vi "plunge_mode_scaled.vi"() -> ()   [LabVIEW 2019]
uses:
  <userlib>/Nanonis Prog Interface V5/Nanonis Prog Interface.lvlib
  <userlib>/Haptic Prog Interface/Haptic Prog Interface.lvlib
panel:
  out "Zthresh (m)":dbl
  in  "Fine Adj":dbl=1.0
  in  "Rough Adj.":dbl
  out "force":dbl
  out "Z Write (m) 2":dbl
  in  "Z Write?":bool
  in  "Save":bool
  in  "# Sample Points":i32=16384
  out "Signal value":sgl format="%#_6p"
  out "Z Write (m)":dbl
  in  "Upper Limit (mm)":dbl=50.0
  in  "Lower Limit (mm)":dbl=-40.0
  in  "Upper Limit (nm)":dbl=80.0
  in  "Lower Limit (nm)":dbl=79.0
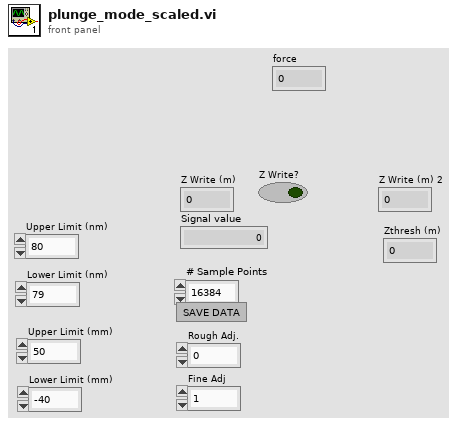
[diagram p1: front panel]
types:
  T1 = cluster{"Fx (N)":dbl, "Fy (N)":dbl, "Fz (N)":dbl}
  T2 = cluster{"x (mm)":dbl, "y (mm)":dbl, "z (mm)":dbl}
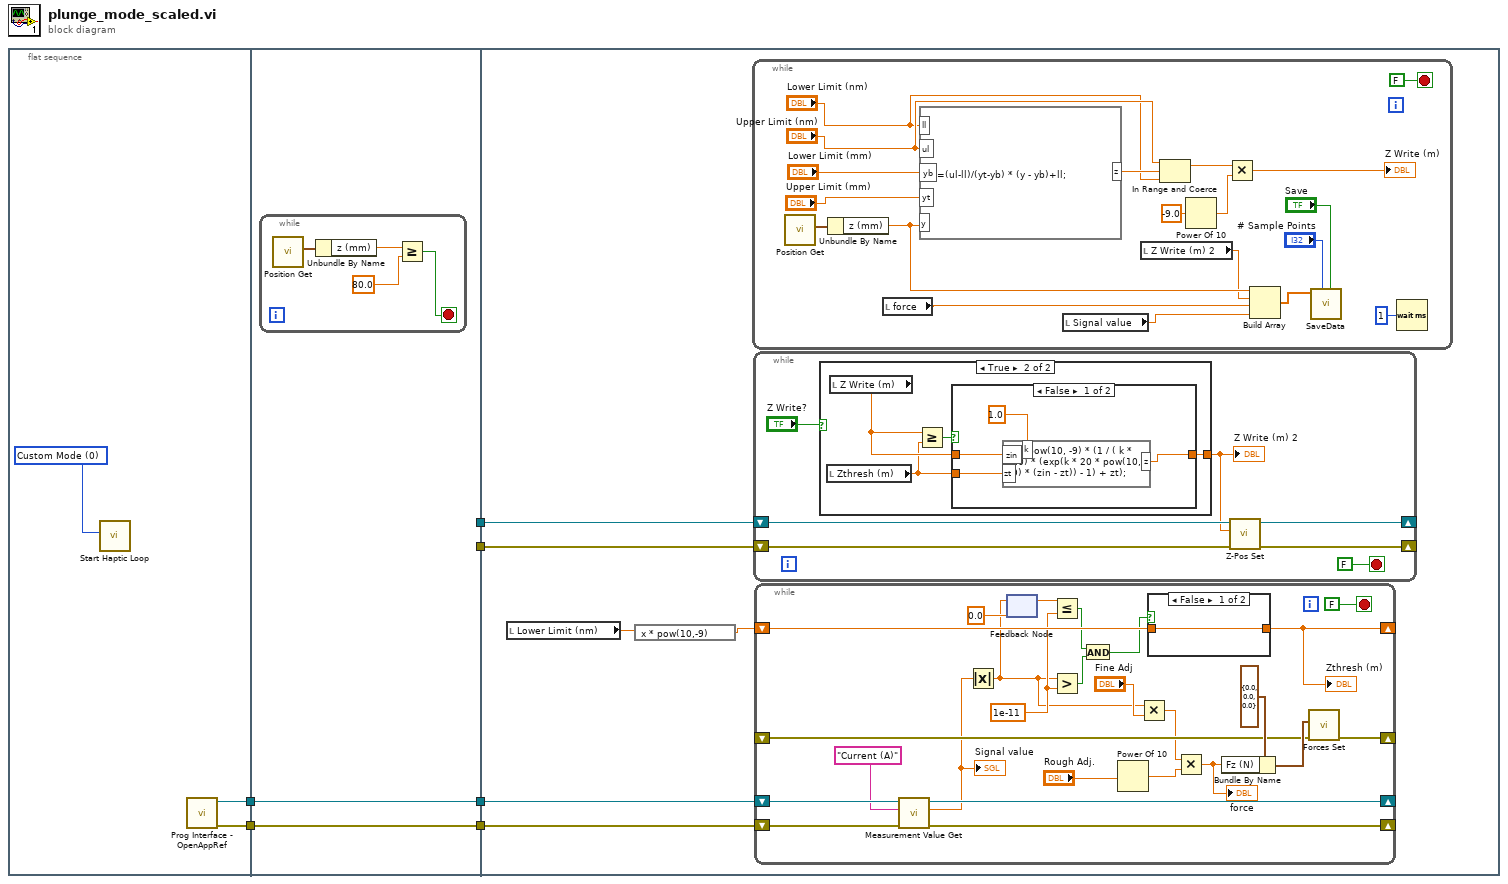
[diagram p0: block diagram]
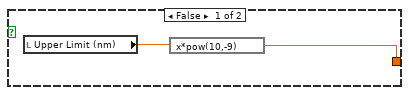
[diagram p2: hidden frame]
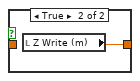
[diagram p4: hidden frame]
diagram:
  n1 = flat-sequence {
    tunnel: [w9] -> w6
    tunnel: [w8] -> w3
    tunnel: [w11] -> w5
    tunnel: [w10] -> w4
    tunnel: [w11] -> w2
    tunnel: [w10] -> w1
    tunnel: w3 -> [w10]
    tunnel: w6 -> [w11]
    tunnel: w5 -> [w21]
    tunnel: w4 -> [w20]
    tunnel: w2 -> [w19]
    tunnel: w1 -> [w18]
    frame #0 {
      w7 = u16 0 items=["Custom Mode", "Read Mode", "Write Mode"] ("Mode Selection")
      n2 = call <userlib>:"Start Haptic Loop.vi"("Mode Selection"=w7) -> ()  [unwired: 10 in, 1 out]
      n3 = call <userlib>:"Prog Interface - OpenAppRef.vi"() -> ("Error out"=w8:errorcluster, "Application reference"=w9:refnum<vi>)  [unwired: 6 in]
    }
    frame #1 {
      n4 = while {
        stop <- w14 stop-if-true
        n5 = call <userlib>:"Position Get.vi"() -> ("Position"=w13:T2)  [unwired: 10 in, 1 out]
        n6 = Unbundle By Name(w13) -> ("z (mm)"=w12:dbl)
        n7 = Greater Or Equal?(x=w12, y=80.0) -> (x >= y?=w14:bool)
      }
    }
    frame #2 {
      n8 = local read "Lower Limit (nm)"() -> (w17:dbl)
      n9 = expression code="x * pow(10,-9)"(w17) -> (w16:dbl)
      n10 = while {
        stop <- FALSE stop-if-true
        n11 = call <userlib>:"Position Get.vi"() -> ("Position"=w71:T2)  [unwired: 10 in, 1 out]
        n12 = Unbundle By Name(w71) -> ("z (mm)"=w70:dbl)
        n13 = local read "force"() -> (w68:dbl)
        n14 = formula code="z =(ul-ll)/(yt-yb) * (y - yb)+ll;"("ll"="Lower Limit (nm)", "ul"="Upper Limit (nm)", "yb"="Lower Limit (mm)", "yt"="Upper Limit (mm)", "y"=w70) -> ("z"=w81:dbl)
        n15 = local read "Signal value"() -> (w74:sgl)
        n16 = local read "Z Write (m) 2"() -> (w69:dbl)
        n17 = In Range and Coerce(upper limit="Upper Limit (nm)", x=w81, lower limit="Lower Limit (nm)") -> (coerced(x)=w77:dbl)  [unwired: 1 out]
        n18 = Power Of 10(x=-9.0) -> (10^x=w82:dbl)
        n19 = Multiply(x=w77, y=w82) -> (x*y=→"Z Write (m)":dbl)
        n20 = Build Array(w70, w69, w68, w74) -> (w73:dbl[])
        n21 = call "SaveData.vi"("Save"="Save", "# Sample Points"="# Sample Points", "Data"=w73) -> ()  [unwired: 9 in]
        n22 = Wait (ms)(milliseconds to wait=u32 1) -> ()  [unwired: 1 out]
      }
      n23 = while {
        shift-right: [w24] -> _
        shift-left: w19 -> [w26]
        shift-right: [w23] -> _
        shift-left: w18 -> [w25]
        stop <- FALSE stop-if-true
        n24 = case shown="True" "Z Write?" {
          tunnel: [w29 w33] -> w22
          frame False {
            n25 = local read "Upper Limit (nm)"() -> (w30:dbl)
            n26 = expression code="x*pow(10,-9)"(w30) -> (w29:dbl)
          }
          frame True {
            n27 = local read "Zthresh (m)"() -> (w31:dbl)
            n28 = local read "Z Write (m)"() -> (w32:dbl)
            n29 = Greater Or Equal?(x=w32, y=w31) -> (x >= y?=w34:bool)
            n30 = case shown="False" w34 {
              tunnel: w32 -> [w38 w39]
              tunnel: [w36 w39] -> w33
              tunnel: w31 -> [w37 _]
              frame False {
                n31 = formula code="z =pow(10, -9) * (1 / ( k * 20) * (exp(k * 20 * pow(10, 9) * (zin - zt)) - 1) + zt);"("zt"=w37, "zin"=w38, "k"=1.0 ("input variable")) -> ("z"=w36:dbl)
              }
              frame True {
              }
            }
          }
        }
        "Z Write (m) 2" <- w22
        n32 = call <userlib>:"Z-Pos Set.vi"("error in (no error)"=w25, "Z position (m)"=w22, "Application ref in"=w26) -> ("error out"=w23:errorcluster, "Application ref out"=w24:refnum<vi>)  [unwired: 7 in]
      }
      n33 = while {
        shift-right: [w61] -> _
        shift-left: w21 -> [w63]
        shift-right: [w60] -> _
        shift-left: w20 -> [w62]
        shift-right: [w56] -> _
        shift-left: _ -> [w55]
        shift-right: [w50] -> _
        shift-left: w16 -> [w49]
        stop <- FALSE stop-if-true
        w44 = 1e-11 ("y")
        n34 = call <userlib>:"Measurement Value Get.vi"("error in (no error)"=w62, "Signal Name"="Current (A)", "Application ref in"=w63) -> ("error out"=w60:errorcluster, "Measurement value"=w41:sgl, "Application ref out"=w61:refnum<vi>)  [unwired: 5 in]
        "Signal value" <- w41
        n35 = Absolute Value(x=w41) -> (abs(x)=w40:sgl)
        n36 = feedback-in #1(w40) -> ()
        n37 = feedback #1(sgl 0.0 ("Measurement value")) -> (w45:sgl)
        n38 = Less Or Equal?(x=w45, y=w44) -> (x <= y?=w46:bool)
        n39 = Greater?(x=w40, y=w44) -> (0:w43:bool)
        n40 = And(x=w46, y=w43) -> (x .and. y?=w48:bool)
        n41 = Power Of 10(x="Rough Adj.") -> (10^x=w53:dbl)
        n42 = Multiply(x=w40, y="Fine Adj") -> (x*y=w52:dbl)
        n43 = case shown="False" w48 {
          tunnel: [w65 w66] -> w50
          tunnel: w49 -> [w65 _]
          frame False {
          }
          frame True {
            n44 = local read "Z Write (m)"() -> (w66:dbl)
          }
        }
        "Zthresh (m)" <- w50
        n45 = Multiply(x=w52, y=w53) -> (x*y=w42:dbl)
        "force" <- w42
        n46 = Bundle By Name(cluster=T1 {"Fx (N)"=0.0, "Fy (N)"=0.0, "Fz (N)"=0.0} ("Force (N)"), "Fz (N)"=w42) -> (w57:T1)
        n47 = call <userlib>:"Forces Set.vi"("error in (no error)"=w55, "Force (N)"=w57) -> ("error out"=w56:errorcluster)  [unwired: 9 in]
      }
    }
  }
